vi "UPDATE_DAC_VALUES.vi"(5 "A":u16=2222, 6 "D":u16=2222, 7 "B":u16=2222, 8 "error in (no error)":errorcluster, 9 "LINX Resource in":T1, 10 "I2C Channel (0)":u8, 11 "C":u16=2222) -> (0 "error out":errorcluster, 3 "LINX Resource out":T1)   [LabVIEW 2018]
uses:
  <vilib>/MakerHub/LINX/Private/Type Defs/LINX Ref.ctl
  <vilib>/MakerHub/LINX/Private/Type Defs/Platform.ctl
  <vilib>/MakerHub/LINX/Private/Type Defs/Interface.ctl
  <vilib>/MakerHub/LINX/Private/Device/Type Defs/LINX Device Config.ctl
  <vilib>/MakerHub/LINX/Private/Device/Type Defs/TCP Config.ctl
  <vilib>/MakerHub/LINX/Private/Device/Type Defs/Channels.ctl
  <vilib>/MakerHub/LINX/Private/Local IO/LinxI2cWrite.vi
  <vilib>/MakerHub/LINX/Public/Utilities/Check Channel.vi
  <vilib>/MakerHub/LINX/Private/Utilties/Generate Error.vi
  <vilib>/MakerHub/LINX/LMH-LINX.lvlib
  <vilib>/MakerHub/LINX/Private/Device/Device.lvlib
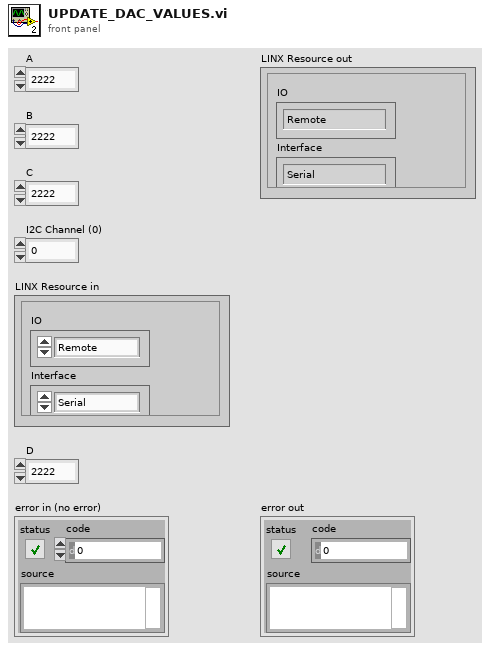
[diagram p1: front panel]
types:
  T1 = typedef "LMH-LINX.lvlib/LINX Ref.ctl" = cluster{"IO":T2, "Interface":T3, "LINX Device Config":T4}
  T2 = typedef "LMH-LINX.lvlib/Platform.ctl" = enum16{"Remote", "Local"}
  T3 = typedef "LMH-LINX.lvlib/Interface.ctl" = enum16{"Serial", "TCP"}
  T4 = typedef "LMH-LINX.lvlib/Device.lvlib/LINX Device Config.ctl" = cluster{"Interface":T3, "COM Port":refnum<visa-resource-name>, "TCP Configuration":T5, "Device Family":u8, "Device ID":u8, "Device Name":string, "TCP Ref":refnum<k5>, "Channels":T6}
  T5 = typedef "LMH-LINX.lvlib/Device.lvlib/TCP Config.ctl" = cluster{"IP Address":string, "Port":u16}
  T6 = typedef "LMH-LINX.lvlib/Channels.ctl" = cluster{"DI":u8[], "DO":u8[], "AI":u8[], "AO":u8[], "PWM":u8[], "QE":u8[], "UART":u8[], "I2C 2":u8[], "SPI":u8[], "CAN":u8[], "Servo":u8[], "AI Ref (V)":dbl, "AI Resolution (Bits)":u8, "AO Ref (V)":dbl, "AO Resolution (Bits)":u8}
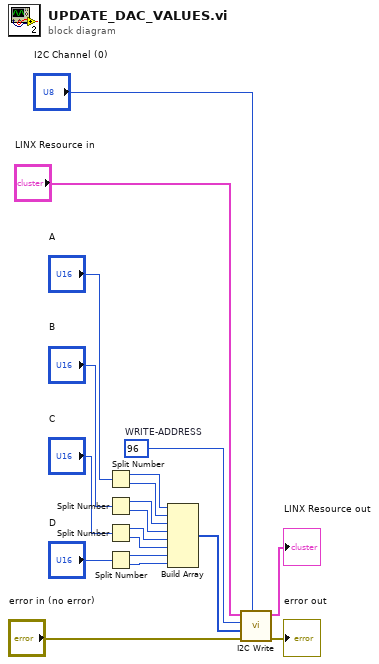
[diagram p0: block diagram]
diagram:
  w16 = u8 96  # WRITE-ADDRESS
  n1 = Split Number(x="A") -> (hi(x)=w9:u8, lo(x)=w8:u8)
  n2 = Split Number(x="B") -> (hi(x)=w7:u8, lo(x)=w6:u8)
  n3 = Split Number(x="C") -> (hi(x)=w5:u8, lo(x)=w4:u8)
  n4 = Split Number(x="D") -> (hi(x)=w3:u8, lo(x)=w14:u8)
  n5 = Build Array(w9, w8, w7, w6, w5, w4, w3, w14) -> (w15:u8[])
  n6 = call <vilib>:"I2C Write.vi"("I2C Channel"="I2C Channel (0)", "Error In"="error in (no error)", "Data"=w15, "I2C Slave Address (0)"=w16, "LINX Resource"="LINX Resource in") -> ("Error Out"=→"error out":errorcluster, "LINX Resource"=→"LINX Resource out":T1)  [unwired: 5 in]
